vi "Delete Tree.vi"(8 "error in (no error)":errorcluster, 11 "Base Tree in":refnum<class "Base Tree.lvclass">) -> (0 "error out":errorcluster)   [LabVIEW 2017, in "Browser Core.lvlib" / "Base Tree.lvclass"]
doc: "Use this as the destructor for the tree object"
uses:
  Base Tree.lvclass
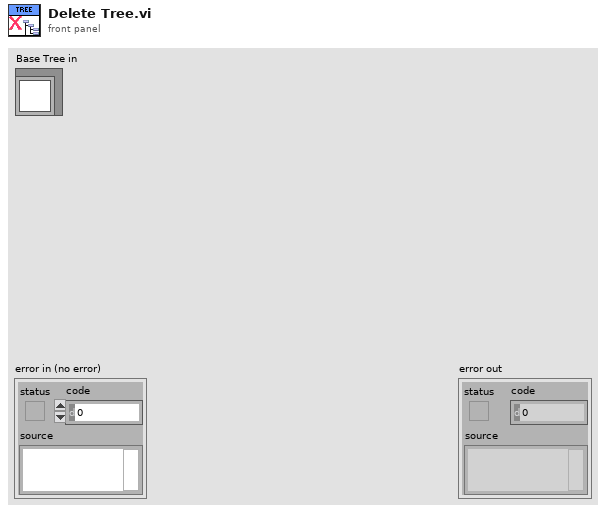
[diagram p1: front panel]
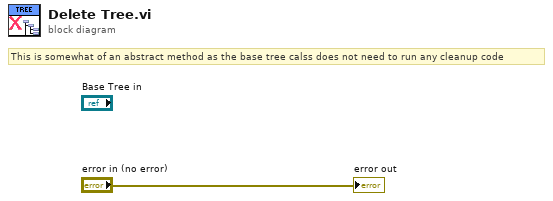
[diagram p0: block diagram]
diagram:
  # "This is somewhat of an abstract method as the base tree calss does not need to run any cleanup code"
  "error out" <- "error in (no error)"
